vi "SPI Master [FPGA].vi"() -> ()   [LabVIEW 2019]
uses:
  <vilib>/Platform/TimedLoop/XDataNode/timing_clust.ctl
  <vilib>/Platform/TimedLoop/XDataNode/nitl_modes.ctl
  <vilib>/Platform/TimedLoop/XDataNode/wakeup.ctl
  SPI Master State.ctl
  <vilib>/rvi/Emulation/niFpgaSctlEmulationGetInTimedLoop.vi
  <vilib>/rvi/Emulation/niFpgaEmulationReportErrorSimple.vi
  <vilib>/rvi/Emulation/niFpgaGetClockAttributes.vi
  <vilib>/rvi/Emulation/niFpgaCriticalErrorInLSC.vi
  <vilib>/Platform/TimedLoop/XDataNode/XDataNode.xnode
  <vilib>/Platform/TimedLoop/XDataNode/XDNodeRunTimeDep.lvlib
  <vilib>/rvi/DataTransferAndStorage/Container/XNode/niFpgaContainer.xnode
  <vilib>/rvi/interface/RandomDataEmulation/nirviRandomDataFpgaReadWriteTemplate.vi
panel:
  in  "Data Length":u8
  in  "HCP-1":u8
  out "Data Out":u32
  in  "Data In":u32
  in  "TX":bool
  in  "CPOL":bool
  in  "CPHA":bool
  in  "RESET":bool
  out "_SS":bool
  out "SCLK":bool
  out "MOSI":bool
  in  "MISO":bool
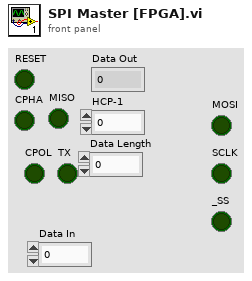
[diagram p1: front panel]
types:
  T1 = typedef "XDNodeRunTimeDep.lvlib/timing_clust.ctl" = cluster{"Expected End [f-1]":u64, "Actual End [f-1]":u64, "Finished Late? [f-1]":bool, "Expected End [i-1]":u64, "Actual End [i-1]":u64, "Finished Late? [i-1]":bool, "Expected Start [i]":u64, "Actual Start [i]":u64, "Expected Start [f]":u64, "Actual Start [f]":u64, "Source Name":string, "Structure Name":string, "Period":i64, "Deadline":i64, "Offset":i64, "Start":i64, "Priority":i32, "Timeout":i32, "Mode":T2, "Wakeup Reason":T3, "Error":errorcluster, "Source Type":string, "Secondary Source Type":string, "Global End Time":u64, "Global Start Time":u64, "Frame Duration":u64, "Iteration Duration":u64, "Assigned CPU":i32, "I/O Scan Engine Mode":u32}
  T2 = typedef "XDNodeRunTimeDep.lvlib/nitl_modes.ctl" = enum32{"No Change", "Process missed periods, maintain original phase", "Discard missed periods, maintain original phase", "Process missed periods, ignore original phase", "Discard missed periods, ignore original phase"}
  T3 = typedef "XDNodeRunTimeDep.lvlib/wakeup.ctl" = enum32{"Normal", "Aborted", "Asynchronous wakeup", "Timing source error", "Timed loop error", "Timeout"}
  T4 = typedef "SPI Master State.ctl" = enum8{"RESET", "Wait for TX", "Assert MOSI", "Toggle SCLK", "Latch MISO and Toggle SCLK", "Assert MOSI and Toggle SCLK"}
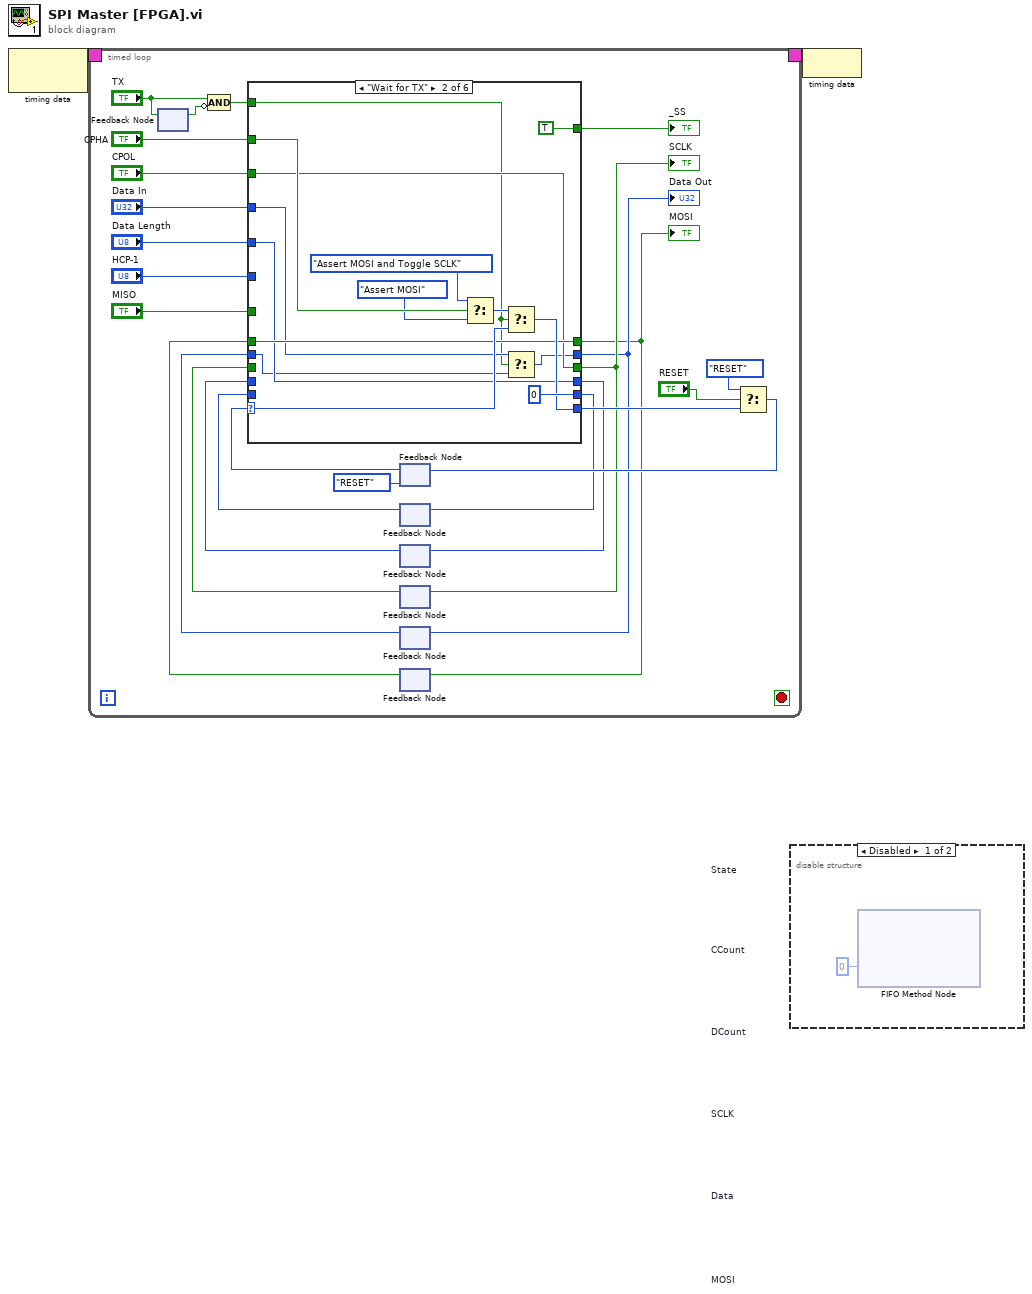
[diagram p0: block diagram]
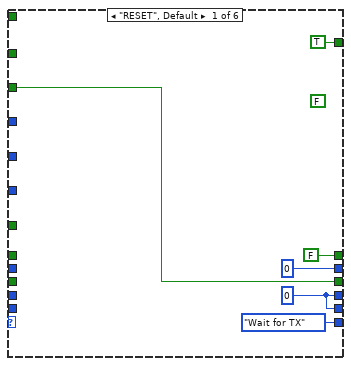
[diagram p3: hidden frame]
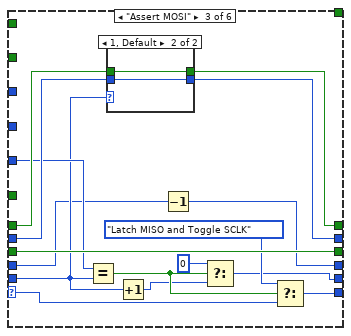
[diagram p4: hidden frame]
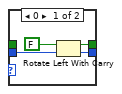
[diagram p5: hidden frame]
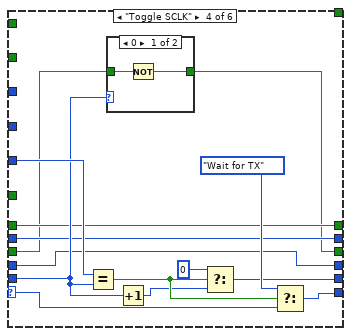
[diagram p6: hidden frame]
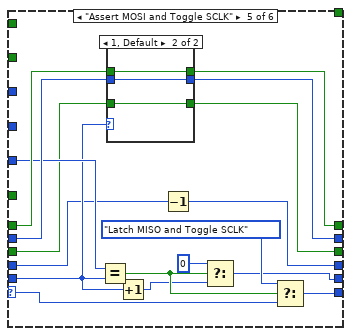
[diagram p8: hidden frame]
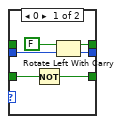
[diagram p9: hidden frame]
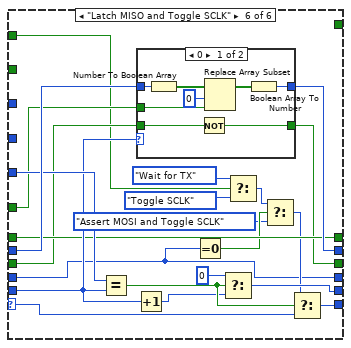
[diagram p10: hidden frame]
diagram:
  n1 = node-c288() -> (w2:T1)  [unwired: 1 in]
  n2 = timed-loop {
    timing: w2 -> [_]
    timing-out: [_] -> w1
    stop <- _ stop-if-true
    n3 = feedback #1() -> (w21:bool)  [unwired: 1 in]
    n4 = feedback-in #1("TX") -> ()
    n5 = Compound Arithmetic op=AND("TX", invert w21) -> (w8:bool)
    n6 = feedback #2 "State"(SPI_Master_State."RESET") -> (w27:T4)
    n7 = feedback #3 "CCount"() -> (w18:u8)  [unwired: 1 in]
    n8 = feedback #4 "DCount"() -> (w17:u8)  [unwired: 1 in]
    n9 = feedback #5 "SCLK"() -> (w13:bool)  [unwired: 1 in]
    n10 = feedback #6 "Data"() -> (w10:u32)  [unwired: 1 in]
    n11 = feedback #7 "MOSI"() -> (w5:bool)  [unwired: 1 in]
    n12 = case shown="\"Wait for TX\"" w27 {
      selector: w27 -> [_ w46 w58 w83 w99 w132]
      tunnel: [SPI_Master_State."Wait for TX" w45 w59 w84 w100 w133] -> w25
      tunnel: w8 -> [_ w37 _ _ _ _]
      tunnel: [w33 u8 0 w52 w77 w93 w127] -> w20
      tunnel: [w33 w40 w50 w76 w91 w115] -> w19
      tunnel: w18 -> [_ _ w55 w80 w96 w130]
      tunnel: w17 -> [_ _ w51 w76 w92 w115]
      tunnel: [TRUE ("MOSI") TRUE ("MOSI") _ _ _ _] -> w16
      tunnel: "CPHA" -> [_ w47 _ _ _ w121]
      tunnel: [w31 w39 w61 w72 w89 w123] -> w12
      tunnel: "CPOL" -> [w31 w39 _ _ _ _]
      tunnel: w13 -> [_ _ w61 w73 w90 w124]
      tunnel: "Data In" -> [_ w38 _ _ _ _]
      tunnel: [u32 0 ("Data In") w36 w64 w75 w104 w135] -> w7
      tunnel: w10 -> [_ w35 w65 w75 w105 w136]
      tunnel: "HCP-1" -> [_ _ w60 w85 w101 w134]
      tunnel: "MISO" -> [_ _ _ _ _ w125]
      tunnel: "Data Length" -> [_ w40 _ _ _ _]
      tunnel: [FALSE ("msb carry out") w41 w63 w74 w103 w126] -> w6
      tunnel: w5 -> [_ w41 w62 w74 w102 w126]
      frame "RESET", Default {
        (unwired) FALSE ("msb carry out")
        w33 = u8 0
      }
      frame "Wait for TX" {
        n13 = Select(t=SPI_Master_State."Assert MOSI and Toggle SCLK", s=w47, f=SPI_Master_State."Assert MOSI" ("t")) -> (s? t:f=w42:T4)
        n14 = Select(t=w42, s=w37, f=w46) -> (s? t:f=w45:T4)
        n15 = Select(t=w38, s=w37, f=w35) -> (s? t:f=w36:u32)
      }
      frame "Assert MOSI" {
        n16 = Equal?(x=w60, y=w55) -> (x = y?=w56:bool)
        n17 = case shown="1, Default" w55 {
          tunnel: w65 -> [w68 w70]
          tunnel: [w67 w70] -> w64
          tunnel: [w66 w71] -> w63
          tunnel: w62 -> [_ w71]
          frame 0 {
            n18 = Rotate Left With Carry(2:w68, 3:FALSE ("carry")) -> (0:w67:u32, 1:w66:bool)
          }
          frame 1, Default {
          }
        }
        n19 = Increment(x=w55) -> (x+1=w54:u8)
        n20 = Decrement(x=w51) -> (x-1=w50:u8)
        n21 = Select(t=u8 0, s=w56, f=w54) -> (s? t:f=w52:u8)
        n22 = Select(t=SPI_Master_State."Latch MISO and Toggle SCLK", s=w56, f=w58) -> (s? t:f=w59:T4)
      }
      frame "Toggle SCLK" {
        n23 = Equal?(x=w85, y=w80) -> (x = y?=w81:bool)
        n24 = case shown="0" w80 {
          tunnel: w73 -> [w87 w88]
          tunnel: [w86 w88] -> w72
          frame 0 {
            n25 = Not(x=w87) -> (.not. x?=w86:bool)
          }
          frame 1, Default {
          }
        }
        n26 = Increment(x=w80) -> (x+1=w79:u8)
        n27 = Select(t=u8 0, s=w81, f=w79) -> (s? t:f=w77:u8)
        n28 = Select(t=SPI_Master_State."Wait for TX", s=w81, f=w83) -> (s? t:f=w84:T4)
      }
      frame "Assert MOSI and Toggle SCLK" {
        n29 = Equal?(x=w101, y=w96) -> (x = y?=w97:bool)
        n30 = case shown="1, Default" w96 {
          tunnel: w105 -> [w110 w113]
          tunnel: [w109 w113] -> w104
          tunnel: [w108 w114] -> w103
          tunnel: w102 -> [_ w114]
          tunnel: w90 -> [w107 w112]
          tunnel: [w106 w112] -> w89
          frame 0 {
            n31 = Not(x=w107) -> (.not. x?=w106:bool)
            n32 = Rotate Left With Carry(2:w110, 3:FALSE ("carry")) -> (0:w109:u32, 1:w108:bool)
          }
          frame 1, Default {
          }
        }
        n33 = Increment(x=w96) -> (x+1=w95:u8)
        n34 = Decrement(x=w92) -> (x-1=w91:u8)
        n35 = Select(t=u8 0, s=w97, f=w95) -> (s? t:f=w93:u8)
        n36 = Select(t=SPI_Master_State."Latch MISO and Toggle SCLK", s=w97, f=w99) -> (s? t:f=w100:T4)
      }
      frame "Latch MISO and Toggle SCLK" {
        n37 = Equal?(x=w134, y=w130) -> (x = y?=w131:bool)
        n38 = Increment(x=w130) -> (x+1=w129:u8)
        n39 = case shown="0" w130 {
          tunnel: w136 -> [w144 w146]
          tunnel: [w139 w146] -> w135
          tunnel: w125 -> [w142 _]
          tunnel: w124 -> [w138 w145]
          tunnel: [w137 w145] -> w123
          frame 0 {
            n40 = Number To Boolean Array(number=w144) -> (Boolean array=w143:bool[])
            n41 = Not(x=w138) -> (.not. x?=w137:bool)
            n42 = Replace Array Subset(array=w143, new element=w142, index=0) -> (w140:bool[])
            n43 = Boolean Array To Number(Boolean array=w140) -> (number=w139:u32)
          }
          frame 1, Default {
          }
        }
        n44 = Equal To 0?(x=w115) -> (x = 0?=w122:bool)
        n45 = Select(t=u8 0, s=w131, f=w129) -> (s? t:f=w127:u8)
        n46 = Select(t=SPI_Master_State."Wait for TX", s=w121, f=SPI_Master_State."Toggle SCLK" ("t")) -> (s? t:f=w117:T4)
        n47 = Select(t=w117, s=w122, f=SPI_Master_State."Assert MOSI and Toggle SCLK" ("t")) -> (s? t:f=w119:T4)
        n48 = Select(t=w119, s=w131, f=w132) -> (s? t:f=w133:T4)
      }
    }
    "SCLK" <- w12
    "_SS" <- w16
    "MOSI" <- w6
    "Data Out" <- w7
    n49 = feedback-in #3(w20) -> ()
    n50 = feedback-in #4(w19) -> ()
    n51 = feedback-in #5(w12) -> ()
    n52 = feedback-in #6(w7) -> ()
    n53 = feedback-in #7(w6) -> ()
    n54 = Select(t=SPI_Master_State."RESET", s="RESET", f=w25) -> (s? t:f=w26:T4)
    n55 = feedback-in #2(w26) -> ()
  }
  n56 = disable-structure shown="Disabled" {
    frame Disabled {
      n57 = xnode ("FIFO Method Node")("Timeout"=0) -> ()  [unwired: 2 in, 2 out]
    }
    frame Enabled {
    }
  }
  n58 = node-c288(w1) -> ()
